vi "_errorHandler..vi"(8 "error in (no error)":errorcluster, 9 "Additional Text":string, 10 "Error Type":T1=enum."Unexpected Token", 11 "JSON Parser In":refnum<class "tJSONParser.lvclass">=refnum) -> (0 "error out":errorcluster, 3 "JSON Parser Out":refnum<class "tJSONParser.lvclass">)   [LabVIEW 2013, in "JSON.lvlib" / "tJSONParser.lvclass"]
doc: "Sets the error code specified by the \"Error Type\" input. Specify any additional text using the \"Additional Text\" input. This text will appear on a new line after the default error text."
uses:
  tJSONParser.lvclass
  _error.ctl
  tJSONParser.lvclass/tJSONParser.ctl
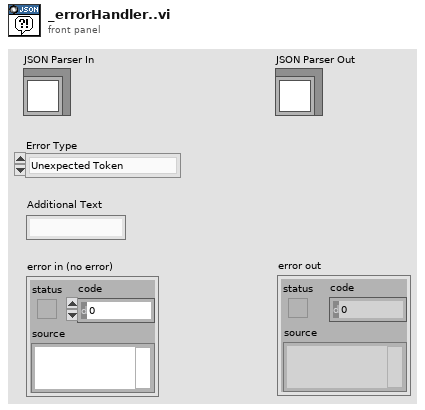
[diagram p1: front panel]
types:
  T1 = typedef "JSON.lvlib/tJSONParser.lvclass/_error.ctl" = enum16{"Missing Object Open", "Missing Pair Separator", "Missing Object End Or Separator", "Missing Pair String", "Unexpected Token", "Missing Array End Or Separator", "Invalid Escape Sequence", "Unexpected End Of File", "Invalid Unicode", "Unexpected End Of Line", "Invalid Numerical Constant"}
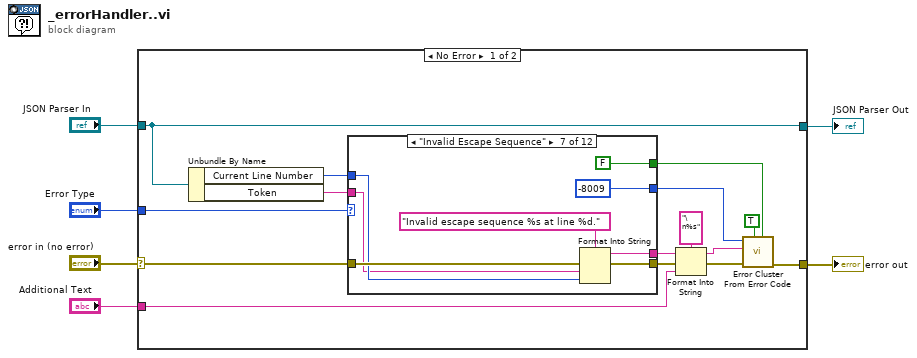
[diagram p0: block diagram]
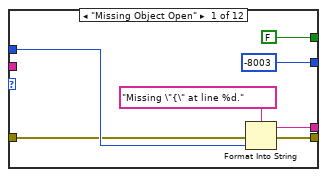
[diagram p2: hidden frame]
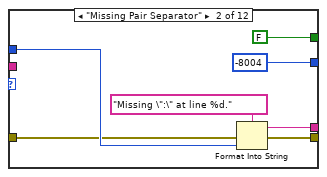
[diagram p3: hidden frame]
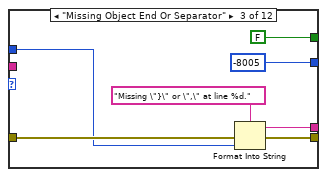
[diagram p4: hidden frame]
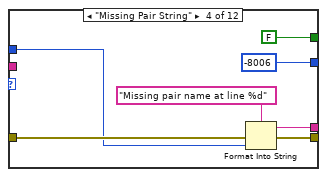
[diagram p5: hidden frame]
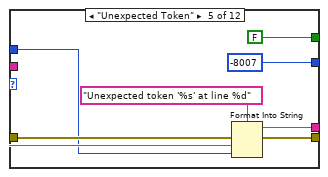
[diagram p6: hidden frame]
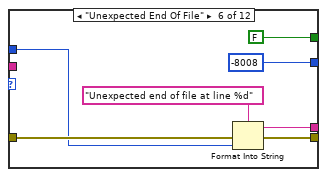
[diagram p7: hidden frame]
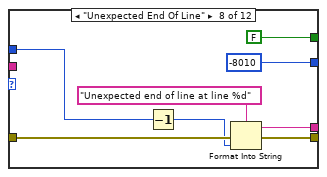
[diagram p8: hidden frame]
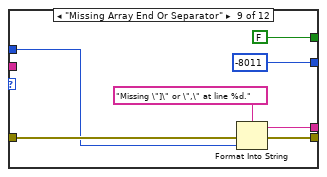
[diagram p9: hidden frame]
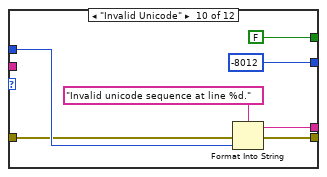
[diagram p10: hidden frame]
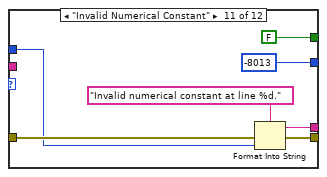
[diagram p11: hidden frame]
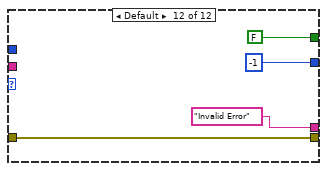
[diagram p12: hidden frame]
diagram:
  n1 = case shown="No Error" "error in (no error)" {
    selector: "error in (no error)" -> [w16 w107]
    tunnel: [w20 w107] -> w5
    tunnel: "Error Type" -> [w21 _]
    tunnel: "Additional Text" -> [w11 _]
    tunnel: "JSON Parser In" -> [w7 w106]
    tunnel: [w7 w106] -> w1
    frame No Error {
      n2 = Unbundle By Name(w7) -> ("Current Line Number"=w8:u32, "Token"=w9:string)
      n3 = case shown="\"Invalid Escape Sequence\"" w21 {
        tunnel: [FALSE FALSE FALSE FALSE FALSE FALSE FALSE FALSE FALSE FALSE FALSE FALSE] -> w18
        tunnel: [-8003 ("error code (0)") -8004 ("error code (0)") -8005 ("error code (0)") -8006 ("error code (0)") -8007 ("error code (0)") -8008 ("error code (0)") -8009 ("error code (0)") -8010 ("error code (0)") -8011 ("error code (0)") -8012 ("error code (0)") -8013 ("error code (0)") -1 ("error code (0)")] -> w17
        tunnel: w16 -> [w22 w29 w38 w45 w53 w59 w68 w75 w83 w88 w98 w103]
        tunnel: [w25 w32 w40 w47 w55 w64 w72 w80 w85 w92 w96 w103] -> w15
        tunnel: [w24 w31 w39 w46 w54 w63 w71 w79 w84 w91 w95 "Invalid Error"] -> w10
        tunnel: w8 -> [w26 w30 w36 w43 w50 w58 w66 w74 w81 w89 w97 _]
        tunnel: w9 -> [_ _ _ _ w51 _ w65 _ _ _ _ _]
        frame "Missing Object Open" {
          n4 = Format Into String(format string="Missing \"{\" at line %d.", error in=w22, w26) -> (resulting string=w24:string, error out=w25:errorcluster)  [unwired: 1 in]
        }
        frame "Missing Pair Separator" {
          n5 = Format Into String(format string="Missing \":\" at line %d.", error in=w29, w30) -> (resulting string=w31:string, error out=w32:errorcluster)  [unwired: 1 in]
        }
        frame "Missing Object End Or Separator" {
          n6 = Format Into String(format string="Missing \"}\" or \",\" at line %d.", error in=w38, w36) -> (resulting string=w39:string, error out=w40:errorcluster)  [unwired: 1 in]
        }
        frame "Missing Pair String" {
          n7 = Format Into String(format string="Missing pair name at line %d", error in=w45, w43) -> (resulting string=w46:string, error out=w47:errorcluster)  [unwired: 1 in]
        }
        frame "Unexpected Token" {
          n8 = Format Into String(format string="Unexpected token '%s' at line %d", error in=w53, w51, w50) -> (resulting string=w54:string, error out=w55:errorcluster)  [unwired: 1 in]
        }
        frame "Unexpected End Of File" {
          n9 = Format Into String(format string="Unexpected end of file at line %d", error in=w59, w58) -> (resulting string=w63:string, error out=w64:errorcluster)  [unwired: 1 in]
        }
        frame "Invalid Escape Sequence" {
          n10 = Format Into String(format string="Invalid escape sequence %s at line %d.", error in=w68, w65, w66) -> (resulting string=w71:string, error out=w72:errorcluster)  [unwired: 1 in]
        }
        frame "Unexpected End Of Line" {
          n11 = Decrement(x=w74) -> (x-1=w73:u32)
          n12 = Format Into String(format string="Unexpected end of line at line %d", error in=w75, w73) -> (resulting string=w79:string, error out=w80:errorcluster)  [unwired: 1 in]
        }
        frame "Missing Array End Or Separator" {
          n13 = Format Into String(format string="Missing \"]\" or \",\" at line %d.", error in=w83, w81) -> (resulting string=w84:string, error out=w85:errorcluster)  [unwired: 1 in]
        }
        frame "Invalid Unicode" {
          n14 = Format Into String(format string="Invalid unicode sequence at line %d.", error in=w88, w89) -> (resulting string=w91:string, error out=w92:errorcluster)  [unwired: 1 in]
        }
        frame "Invalid Numerical Constant" {
          n15 = Format Into String(format string="Invalid numerical constant at line %d.", error in=w98, w97) -> (resulting string=w95:string, error out=w96:errorcluster)  [unwired: 1 in]
        }
        frame Default {
        }
      }
      n16 = Format Into String(format string="\n%s", initial string=w10, error in=w15, w11) -> (resulting string=w13:string, error out=w14:errorcluster)
      n17 = call <vilib>:"Error Cluster From Error Code.vi"("is warning? (False)"=w18, "show call chain? (False)"=TRUE, "error in (no error)"=w14, "error message (\"\")"=w13, "error code (0)"=w17) -> ("error out"=w20:errorcluster)  [unwired: 4 in]
    }
    frame Error {
    }
  }
  "error out" <- w5
  "JSON Parser Out" <- w1
